vi "AIT 1553 - Parse BM Sysdef Tree Messages.vi"(8 "error in":errorcluster, 9 "BM_Messages In":T2[](array[typedef]), 10 "Section Ptr":T1 format="%.0x") -> (0 "error out":errorcluster, 1 "BM_Messages Out":T2[](array[typedef]))   [LabVIEW 2013]
uses:
  <vilib>/NI Veristand/Custom Device API/Custom Device Item Ref.ctl
  Controls/1553_BM_Message.ctl
  Controls/1553 Param.ctl
  Controls and Global/Global.vi
  <vilib>/NI Veristand/Custom Device Tools/Custom Device Utility Library/NI VeriStand - Search for Item by Name.vi
  <vilib>/NI Veristand/Custom Device API/Get Item Property (I32).vi
  <vilib>/NI Veristand/Custom Device API/Get Item Property (Double).vi
  <vilib>/NI Veristand/Custom Device API/Get Item Property (Boolean).vi
  <vilib>/NI Veristand/Custom Device API/Custom Device API.lvlib
  AIT 1553 Custom Device.lvlib
  <vilib>/NI Veristand/Custom Device Tools/Custom Device Utility Library/Custom Device Utility Library.lvlib
panel:
  out "Found":bool[](array[boolean])
  out "Property Names":string[][][](array[string])
  out "Channel Refs":T1[][](array[typedef]) format="%.0x"
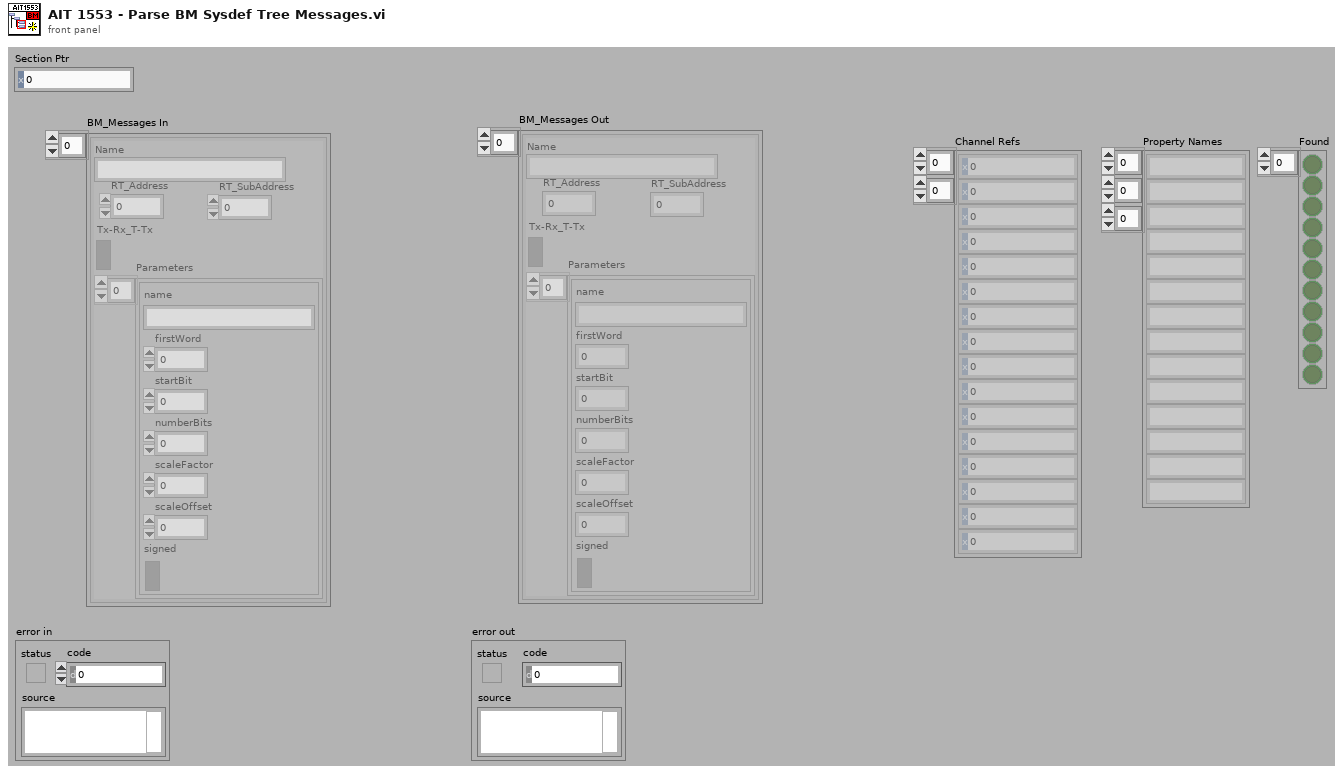
[diagram p1: front panel]
types:
  T1 = typedef "Custom Device API.lvlib/Custom Device Item Ref.ctl" = u64
  T2 = typedef "AIT 1553 Custom Device.lvlib/1553_BM_Message.ctl" = cluster{"RT_Address":u8, "RT_SubAddress":u8, "Tx-Rx_T-Tx":bool, "Parameters":T3[], "Name":string}
  T3 = typedef "AIT 1553 Custom Device.lvlib/1553 Param.ctl" = cluster{"name":string, "firstWord":i32, "startBit":i32, "numberBits":i32, "scaleFactor":dbl, "scaleOffset":dbl, "signed":bool}
  T4 = enum32{"Invalid", "Standard", "Closed", "Hidden", "Minimized", "Maximized"}
  T5 = typedef "Custom Device API.lvlib/Custom Device Item Info.ctl" = cluster{"Name":string, "Is Channel":bool, "GUID":string, "Is Waveform":bool}
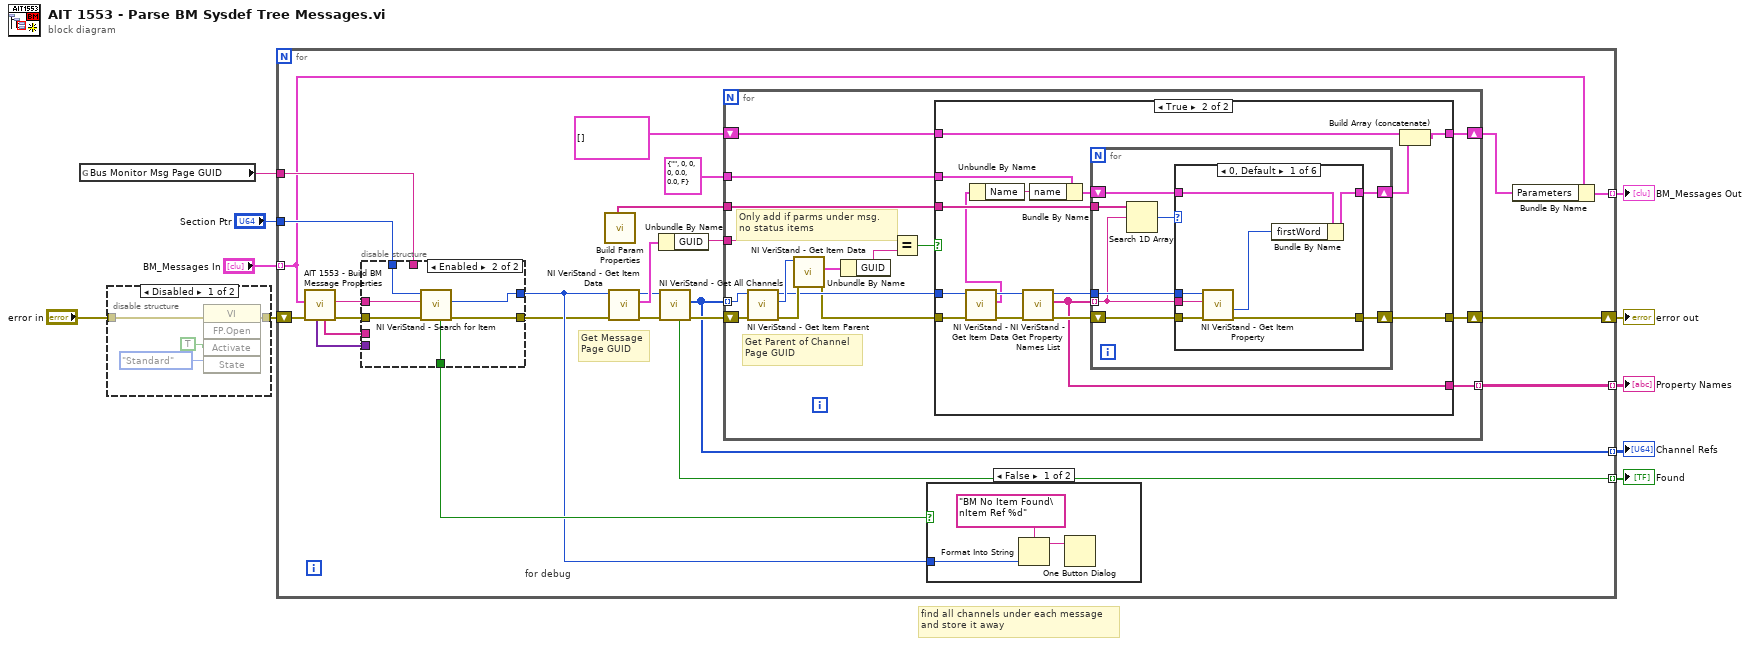
[diagram p0: block diagram]
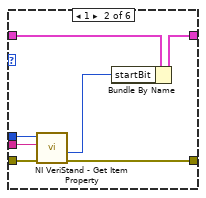
[diagram p5: hidden frame]
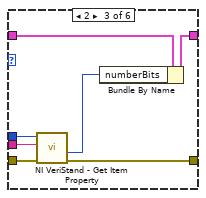
[diagram p6: hidden frame]
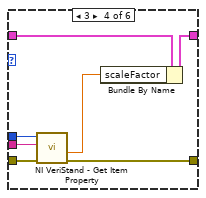
[diagram p7: hidden frame]
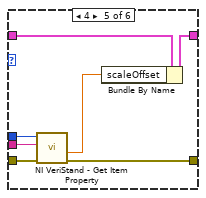
[diagram p8: hidden frame]
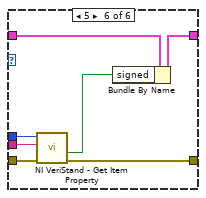
[diagram p9: hidden frame]
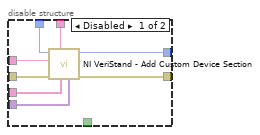
[diagram p10: hidden frame]
diagram:
  # "find all channels under each message\nand store it away"
  n1 = global read "Global.vi" "Bus Monitor Msg Page GUID"() -> (w8:string)
  n2 = disable-structure shown="Disabled" {
    disable-tunnel: "error in" -> [w12 w15]
    disable-tunnel: [w11 w15] -> w4
    frame Disabled {
      n3 = invoke class="VI" method="FP.Open"(error in=w12, "Activate"=TRUE ("Activate?"), "State"=T4."Standard") -> (error out=w11:errorcluster)  [unwired: 2 in, 4 out]
    }
    frame Enabled {
    }
  }
  n4 = for {
    shift-right: [w16] -> w10
    shift-left: w4 -> [w36]
    tunnel: "Section Ptr" -> [w34]
    tunnel: "BM_Messages In" -> [w25] mode=indexing
    tunnel: w8 -> [w35]
    tunnel: [w31] -> w6 mode=indexing
    tunnel: [w29] -> w3 mode=indexing
    tunnel: [w28] -> w2 mode=indexing
    tunnel: [w27] -> w1 mode=indexing
    # "Get Message\nPage GUID"
    # "for debug"
    n5 = call "AIT 1553 - Build BM Message Properties.vi"("error in (no error)"=w36, "BM_Message"=w25) -> ("error out"=w38:errorcluster, "name"=w37:string, "Prop Names"=w39:string[], "Prop Values"=w40:variant[])  [unwired: 5 in, 1 out]
    n6 = disable-structure shown="Enabled" {
      disable-tunnel: w40 -> [w135 _]
      disable-tunnel: w39 -> [w134 _]
      disable-tunnel: w38 -> [w133 w140]
      disable-tunnel: w37 -> [w132 w141]
      disable-tunnel: w35 -> [w131 _]
      disable-tunnel: w34 -> [w130 w139]
      disable-tunnel: [w129 w137] -> w22
      disable-tunnel: [w128 w136] -> w23
      disable-tunnel: [_ w138] -> w30
      frame Disabled {
        n7 = call <vilib>:"NI VeriStand - Add Custom Device Section.vi"("Property Values"=w135, "Property names"=w134, "GUID (Default Section)"=w131, "error in (no error)"=w133, "Section Name"=w132, "Parent Ref in"=w130) -> ("error out"=w129:errorcluster, "Section Ptr"=w128:T1)  [unwired: 2 in, 2 out]
      }
      frame Enabled {
        n8 = call-poly <vilib>:"NI VeriStand - Search for Item.vi"("error in"=w140, "Item Name"=w141, "Section Ref in"=w139) -> ("error out"=w137:errorcluster, "Item Ref"=w136:T1, "Found"=w138:bool)  [unwired: 5 in, 1 out]
      }
    }
    n9 = call "Build Param Properties.vi"() -> ("Prop Names"=w32:string[])  [unwired: 11 in, 8 out]
    n10 = call <vilib>:"NI VeriStand - Get Item Data.vi"("error in (no error)"=w22, "Item Ref in"=w23) -> ("error out"=w21:errorcluster, "Item Info"=w24:T5, "Item Ref out"=w20:T1)  [unwired: 6 in, 1 out]
    n11 = Unbundle By Name(w24) -> ("GUID"=w19:string)
    n12 = call <vilib>:"NI VeriStand - Get All Channels.vi"("error in"=w21, "Section Ref in"=w20) -> ("error out"=w33:errorcluster, "Channel Refs"=w28:T1[], "Found"=w29:bool)  [unwired: 6 in, 1 out]
    n13 = for {
      tunnel: w28 -> [w50] mode=indexing
      tunnel: w32 -> [w59]
      tunnel: [w56] -> w27 mode=indexing
      tunnel: T3 {"name"="", "firstWord"=0, "startBit"=0, "numberBits"=0, "scaleFactor"=0.0, "scaleOffset"=0.0, "signed"=FALSE} ("1553 Parameter") -> [w57]
      tunnel: w19 -> [w47]
      shift-right: [w44] -> w17
      shift-left: T3[] [] -> [w46]
      shift-right: [w58] -> w16
      shift-left: w33 -> [w51]
      # "Only add if parms under msg.\nno status items"
      # "Get Parent of Channel\nPage GUID"
      n14 = call <vilib>:"NI VeriStand - Get Item Parent.vi"("error in (no error)"=w51, "Item Ref in"=w50) -> ("error out"=w55:errorcluster, "Parent Ref"=w54:T1, "Item Ref out"=w49:T1)  [unwired: 6 in, 1 out]
      n15 = call <vilib>:"NI VeriStand - Get Item Data.vi"("error in (no error)"=w55, "Item Ref in"=w54) -> ("error out"=w48:errorcluster, "Item Info"=w53:T5)  [unwired: 6 in, 2 out]
      n16 = Unbundle By Name(w53) -> ("GUID"=w52:string)
      n17 = Equal?(x=w47, y=w52) -> (x = y?=w45:bool)
      n18 = case shown="True" w45 {
        tunnel: w59 -> [_ w76]
        tunnel: [w60 w62] -> w58
        tunnel: w57 -> [_ w72]
        tunnel: [_ w68] -> w56
        tunnel: w49 -> [_ w67]
        tunnel: w48 -> [w60 w66]
        tunnel: w46 -> [w61 w65]
        tunnel: [w61 w63] -> w44
        frame False {
        }
        frame True {
          n19 = call <vilib>:"NI VeriStand - Get Item Data.vi"("error in (no error)"=w66, "Item Ref in"=w67) -> ("error out"=w74:errorcluster, "Item Info"=w69:T5, "Item Ref out"=w73:T1)  [unwired: 6 in, 1 out]
          n20 = Unbundle By Name(w69) -> ("Name"=w70:string)
          n21 = call <vilib>:"NI VeriStand - Get Property Names List.vi"("error in (no error)"=w74, "Item Ref in"=w73) -> ("error out"=w77:errorcluster, "Property Names"=w68:string[], "Item Ref out"=w75:T1)  [unwired: 7 in]
          n22 = Bundle By Name(cluster=w72, "name"=w70) -> (w71:T3)
          n23 = for {
            tunnel: w68 -> [w80] mode=indexing
            tunnel: w76 -> [w85]
            shift-right: [w79] -> w64
            shift-left: w71 -> [w83]
            tunnel: w75 -> [w81]
            shift-right: [w78] -> w62
            shift-left: w77 -> [w82]
            n24 = Search 1D Array(1D array=w85, element=w80) -> (index of element=w84:i32)  [unwired: 1 in]
            n25 = case shown="0, Default" w84 {
              tunnel: w83 -> [w92 w99 w106 w113 w120 w127]
              tunnel: w82 -> [w91 w98 w105 w112 w119 w126]
              tunnel: w81 -> [w90 w97 w104 w111 w118 w125]
              tunnel: w80 -> [w89 w96 w103 w110 w117 w124]
              tunnel: [w87 w94 w101 w108 w115 w122] -> w79
              tunnel: [w86 w93 w100 w107 w114 w121] -> w78
              frame 0, Default {
                n26 = call-poly <vilib>:"NI VeriStand - Get Item Property.vi"("error in (no error)"=w91, "Property Name"=w89, "Item Ref in"=w90) -> ("error out"=w86:errorcluster, "Value"=w88:i32)  [unwired: 5 in, 2 out]
                n27 = Bundle By Name(cluster=w92, "firstWord"=w88) -> (w87:T3)
              }
              frame 1 {
                n28 = call-poly <vilib>:"NI VeriStand - Get Item Property.vi"("error in (no error)"=w98, "Property Name"=w96, "Item Ref in"=w97) -> ("error out"=w93:errorcluster, "Value"=w95:i32)  [unwired: 5 in, 2 out]
                n29 = Bundle By Name(cluster=w99, "startBit"=w95) -> (w94:T3)
              }
              frame 2 {
                n30 = call-poly <vilib>:"NI VeriStand - Get Item Property.vi"("error in (no error)"=w105, "Property Name"=w103, "Item Ref in"=w104) -> ("error out"=w100:errorcluster, "Value"=w102:i32)  [unwired: 5 in, 2 out]
                n31 = Bundle By Name(cluster=w106, "numberBits"=w102) -> (w101:T3)
              }
              frame 3 {
                n32 = call-poly <vilib>:"NI VeriStand - Get Item Property.vi"("error in (no error)"=w112, "Property Name"=w110, "Item Ref in"=w111) -> ("error out"=w107:errorcluster, "Value"=w109:dbl)  [unwired: 5 in, 2 out]
                n33 = Bundle By Name(cluster=w113, "scaleFactor"=w109) -> (w108:T3)
              }
              frame 4 {
                n34 = call-poly <vilib>:"NI VeriStand - Get Item Property.vi"("error in (no error)"=w119, "Property Name"=w117, "Item Ref in"=w118) -> ("error out"=w114:errorcluster, "Value"=w116:dbl)  [unwired: 5 in, 2 out]
                n35 = Bundle By Name(cluster=w120, "scaleOffset"=w116) -> (w115:T3)
              }
              frame 5 {
                n36 = call-poly <vilib>:"NI VeriStand - Get Item Property.vi"("error in (no error)"=w126, "Property Name"=w124, "Item Ref in"=w125) -> ("error out"=w121:errorcluster, "Value"=w123:bool)  [unwired: 5 in, 2 out]
                n37 = Bundle By Name(cluster=w127, "signed"=w123) -> (w122:T3)
              }
            }
          }
          n38 = Build Array (concatenate)(w65, w64) -> (w63:T3[])
        }
      }
    }
    n39 = case shown="False" w30 {
      tunnel: w23 -> [w43 _]
      frame False {
        n40 = Format Into String(format string="BM No Item Found\nItem Ref %d" ("message"), w43) -> (resulting string=w42:string)  [unwired: 2 in, 1 out]
        n41 = One Button Dialog(message=w42) -> ()  [unwired: 1 in, 1 out]
      }
      frame True {
      }
    }
    n42 = Bundle By Name(cluster=w25, "Parameters"=w17) -> (w31:T2)
  }
  "error out" <- w10
  "BM_Messages Out" <- w6
  "Found" <- w3
  "Channel Refs" <- w2
  "Property Names" <- w1
